vi "from string.vi"(8 "error in":errorcluster, 9 "data":string, 10 "version":string, 11 "Daqmx Module configuration in":refnum<class "DAQmx Module Configuration.lvclass">) -> (0 "error out":errorcluster, 3 "Daqmx Module configuration out":refnum<class "DAQmx Module Configuration.lvclass">)   [LabVIEW 2014, in "DAQmx Module Configuration.lvclass"]
doc: "Provides an interface for loading a module configuration from a file or other serialized data source. It is recommended that all children of this class store data in two sets--data required for its own initialization, and any data required for parent initialization--and that each implementation uses the <b>Call Parent Method</b> primitive to de-serialize parent information. As a result, it is expected that every module configuration class calls <b>component configuration.lvclass:From String.vi</b>."
uses:
  DAQmx Module Configuration.lvclass
  Line.ctl
  <vilib>/NI/Tag Bus Module Framework/channel/TBM channel.lvclass
  Measurement Type.ctl
  Parameters.ctl
  DAQmx Module Configuration.lvclass/DAQmx Module Configuration.ctl
  <vilib>/NI/Tag Bus Module Framework/module configuration/TBM module configuration.lvclass
  <vilib>/NI/Configuration Framework/serializable configuration/NISE_CEF_serializable configuration.lvclass
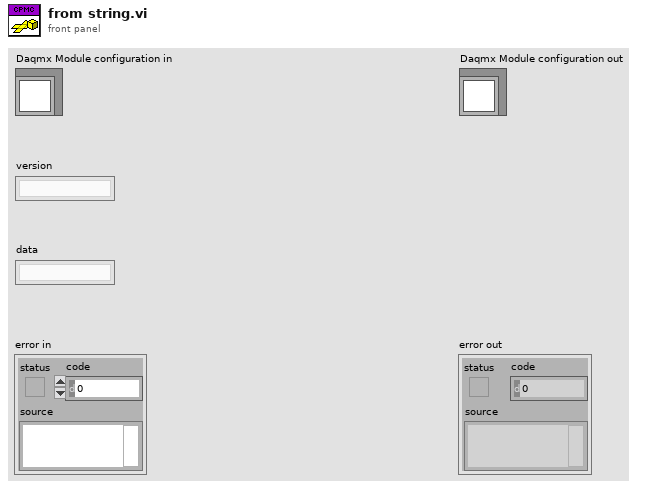
[diagram p1: front panel]
types:
  T1 = typedef "DAQmx Module Configuration.lvclass/Line.ctl" = cluster{"channel":refnum<class "TBM channel.lvclass">, "Physical Channel":string, "Measurement Type":T2, "Parameters":T3}
  T2 = typedef "DAQmx Module Configuration.lvclass/Measurement Type.ctl" = enum16{"Digital Input", "Digital Output", "Voltage Input", "Voltage Output", "Current Input", "Current Output", "RTD", "Thermocouple", "Strain"}
  T3 = typedef "DAQmx Module Configuration.lvclass/Parameters.ctl" = cluster{"Digital Config":cluster{"Invert Lines?":bool}, "Voltage Config":cluster{"Maximum Value (V)":dbl, "Minimum Value (V)":dbl, "in terminal configuration (V)":i32, "out terminal configuration (V)":i32}, "Current Config":cluster{"Maximum Value (A)":dbl, "Minimum Value (A)":dbl, "shunt resistor location":i32, "input terminal configuration (C)":i32, "external shunt resistor value":dbl}, "RTD Config":cluster{"Maximum Value (°C)":dbl, "Minimum Value (°C)":dbl, "resistance configuration":i32, "r0":dbl, "current excitation value":dbl, "rtd type":i32, "current excitation source":i32}, "Thermocouple Config":cluster{"Minimum Value (C)":dbl, "Maximum Value (C)":dbl, "thermocouple type":i32, "cjc source":i32, "cjc value":dbl}, "Strain Config":cluster{"Maximum Value":dbl, "Minimum Value":dbl, "bridge information":cluster{"strain configuration":i32, "lead wire resistance":dbl, "initial bridge voltage":dbl, "voltage excitation source":i32, "voltage excitation value":dbl}, "strain gage information":cluster{"gage factor":dbl, "nominal gage resistance":dbl, "poisson ratio":dbl}}}
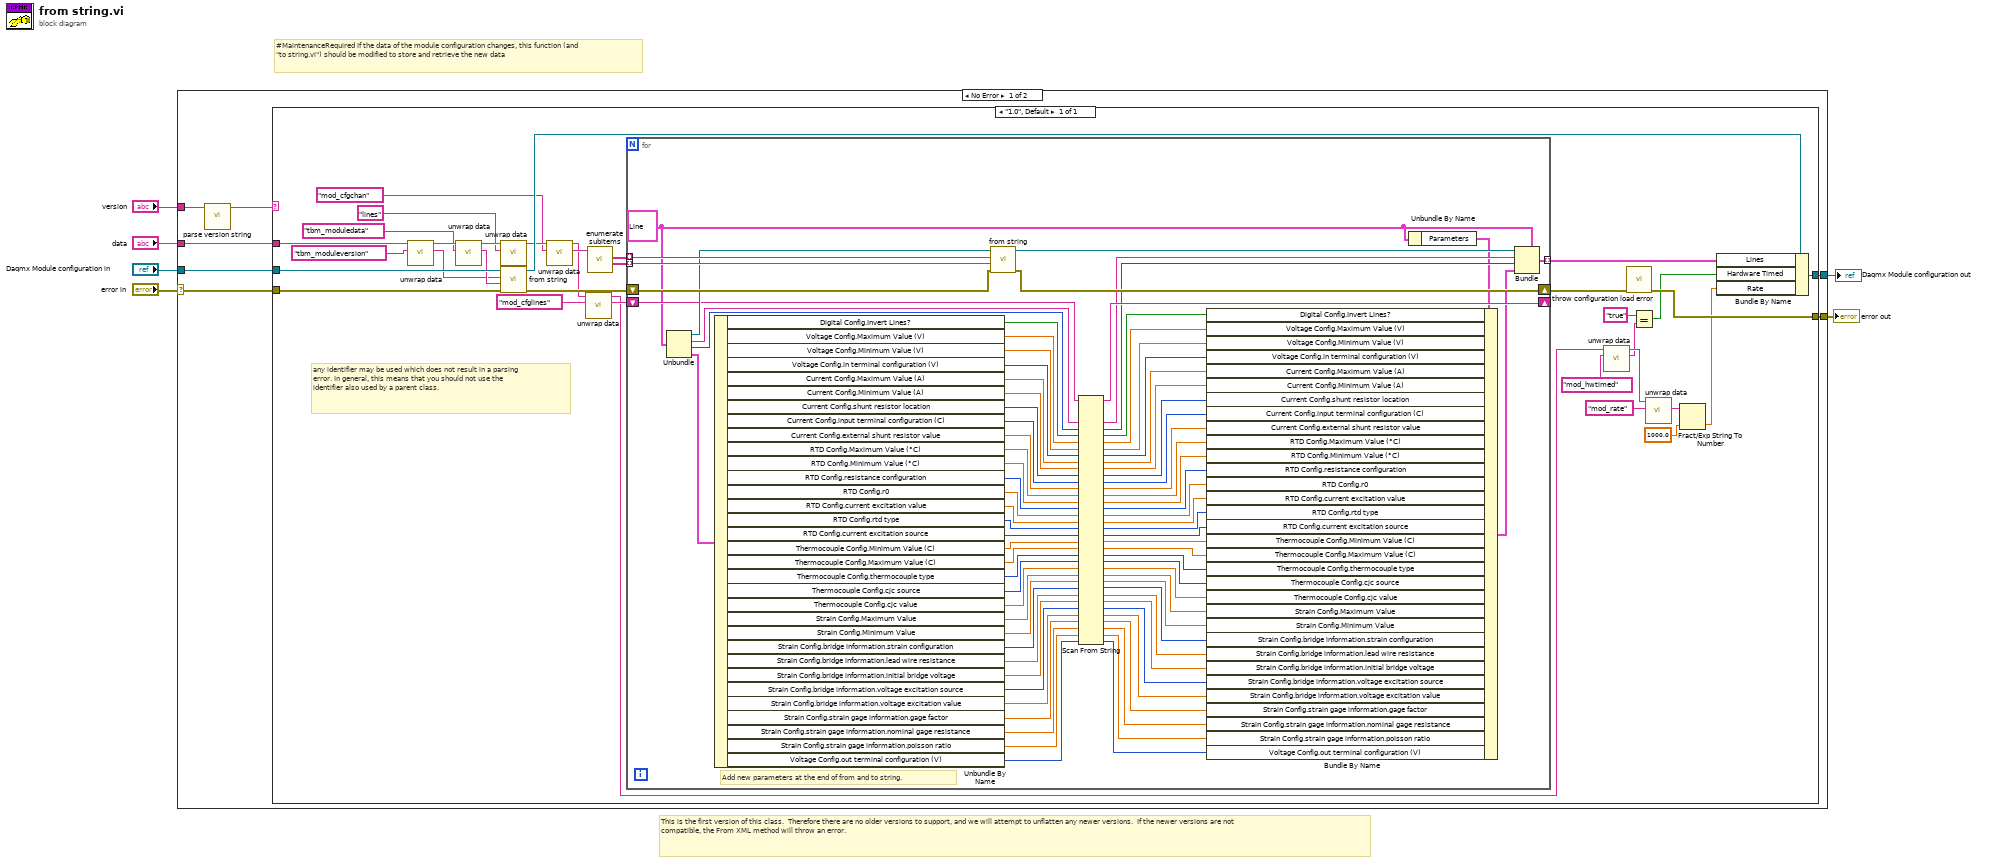
[diagram p0: block diagram]
diagram:
  # "#MaintenanceRequired If the data of the module configuration changes, this function (and \"to string.vi\") should be modified to store and retrieve the new data"
  # "This is the first version of this class.  Therefore there are no older versions to support, and we will attempt to unflatten any newer versions.  If the newer versions are not compatible, the From XML method will throw an error."
  n1 = case shown="No Error" "error in" {
    selector: "error in" -> [w7 w130]
    tunnel: "data" -> [w13 _]
    tunnel: "Daqmx Module configuration in" -> [w12 w129]
    tunnel: [w11 w129] -> w1
    tunnel: [w10 w130] -> w6
    tunnel: "version" -> [w9 _]
    frame No Error {
      n2 = call <vilib>:"parse version string.vi"("full version"=w9) -> ("major.minor version"=w8:string)  [unwired: 7 in, 3 out]
      n3 = case shown="\"1.0\", Default" w8 {
        tunnel: w13 -> [w44]
        tunnel: w7 -> [w43]
        tunnel: w12 -> [w47]
        tunnel: [w35] -> w11
        tunnel: [w46] -> w10
        frame "1.0", Default {
          # "any identifier may be used which does not result in a parsing error. In general, this means that you should not use the identifier also used by a parent class."
          n4 = call <vilib>:"unwrap data.vi"("identifier"="tbm_moduleversion" ("additional identifier"), "data to unwrap"=w44) -> ("unwrapped data"=w39:string, "remaining string"=w45:string)  [unwired: 8 in]
          n5 = call <vilib>:"unwrap data.vi"("identifier"="tbm_moduledata" ("additional identifier"), "data to unwrap"=w45) -> ("unwrapped data"=w41:string, "remaining string"=w38:string)  [unwired: 8 in]
          n6 = call <vilib>:"unwrap data.vi"("identifier"="lines" ("additional identifier"), "data to unwrap"=w38) -> ("remaining string"=w34:string)  [unwired: 8 in, 1 out]
          n7 = call-parent "from string.vi"("error in"=w43, "data"=w41, "version"=w39, "module configuration in"=w47) -> ("error out"=w30:errorcluster, "module configuration out"=w36:refnum<class "DAQmx Module Configuration.lvclass">)  [unwired: 6 in]
          n8 = call <vilib>:"unwrap data.vi"("identifier"="mod_cfgchan", "data to unwrap"=w34) -> ("unwrapped data"=w29:string, "remaining string"=w26:string)  [unwired: 8 in]
          n9 = call <vilib>:"unwrap data.vi"("identifier"="mod_cfglines", "data to unwrap"=w26) -> ("unwrapped data"=w24:string, "remaining string"=w14:string)  [unwired: 8 in]
          n10 = call <vilib>:"enumerate subitems.vi"("data to enumerate"=w29) -> ("associated data"=w31:string[], "discovered subitems"=w32:string[])  [unwired: 8 in, 1 out]
          n11 = for {
            shift-right: [w123] -> w28
            shift-left: w30 -> [w128]
            tunnel: w32 -> [w127] mode=indexing
            tunnel: w31 -> [w126] mode=indexing
            tunnel: [w124] -> w27 mode=indexing
            shift-right: [w95] -> _
            shift-left: w24 -> [w96]
            w51 = T1 {"channel"=refnum, "Physical Channel"="", "Measurement Type"=enum."Digital Input", "Parameters"={"Digital Config"={"Invert Lines?"=FALSE}, "Voltage Config"={"Maximum Value (V)"=5.0, "Minimum Value (V)"=-5.0, "in terminal configuration (V)"=-1, "out terminal configuration (V)"=-1}, "Current Config"={"Maximum Value (A)"=0.02, "Minimum Value (A)"=0.0, "shunt resistor location"=-1, "input terminal configuration (C)"=-1, "external shunt resistor value"=249.0}, "RTD Config"={"Maximum Value (°C)"=100.0, "Minimum Value (°C)"=0.0, "resistance configuration"=2, "r0"=100.0, "current excitation value"=0.0025, "rtd type"=10137, "current excitation source"=10167}, "Thermocouple Config"={"Minimum Value (C)"=0.0, "Maximum Value (C)"=100.0, "thermocouple type"=10072, "cjc source"=10116, "cjc value"=25.0}, "Strain Config"={"Maximum Value"=0.001, "Minimum Value"=-0.001, "bridge information"={"strain configuration"=10183, "lead wire resistance"=0.0, "initial bridge voltage"=0.0, "voltage excitation source"=10200, "voltage excitation value"=2.5}, "strain gage information"={"gage factor"=2.0, "nominal gage resistance"=350.0, "poisson ratio"=0.3}}}} ("Line")
            # "Add new parameters at the end of from and to string."
            n12 = Unbundle(w51) -> ("channel"=w122:refnum<class "TBM channel.lvclass">, "Physical Channel"=w121:string, "Measurement Type"=w97:T2, "Parameters"=w93:T3)
            n13 = Unbundle By Name(w93) -> ("Digital Config.Invert Lines?"=w120:bool, "Voltage Config.Maximum Value (V)"=w119:dbl, "Voltage Config.Minimum Value (V)"=w118:dbl, "Voltage Config.in terminal configuration (V)"=w117:i32, "Current Config.Maximum Value (A)"=w116:dbl, "Current Config.Minimum Value (A)"=w115:dbl, "Current Config.shunt resistor location"=w114:i32, "Current Config.input terminal configuration (C)"=w113:i32, "Current Config.external shunt resistor value"=w111:dbl, "RTD Config.Maximum Value (°C)"=w112:dbl, "RTD Config.Minimum Value (°C)"=w110:dbl, "RTD Config.resistance configuration"=w109:i32, "RTD Config.r0"=w108:dbl, "RTD Config.current excitation value"=w107:dbl, "RTD Config.rtd type"=w106:i32, "RTD Config.current excitation source"=w105:i32, "Thermocouple Config.Minimum Value (C)"=w104:dbl, "Thermocouple Config.Maximum Value (C)"=w103:dbl, "Thermocouple Config.thermocouple type"=w102:i32, "Thermocouple Config.cjc source"=w101:i32, "Thermocouple Config.cjc value"=w100:dbl, "Strain Config.Maximum Value"=w99:dbl, "Strain Config.Minimum Value"=w98:dbl, "Strain Config.bridge information.strain configuration"=w92:i32, "Strain Config.bridge information.lead wire resistance"=w91:dbl, "Strain Config.bridge information.initial bridge voltage"=w90:dbl, "Strain Config.bridge information.voltage excitation source"=w89:i32, "Strain Config.bridge information.voltage excitation value"=w88:dbl, "Strain Config.strain gage information.gage factor"=w87:dbl, "Strain Config.strain gage information.nominal gage resistance"=w86:dbl, "Strain Config.strain gage information.poisson ratio"=w85:dbl, "Voltage Config.out terminal configuration (V)"=w49:i32)
            n14 = call-dynamic "from string.vi"("error in"=w128, "channel data"=w126, "identifier"=w127, "channel in"=w122) -> ("error out"=w123:errorcluster, "channel out"=w125:refnum<class "TBM channel.lvclass">)  [unwired: 6 in]
            n15 = Scan From String(input string=w96, default 1=w121, default 2=w97, default 3=w120, default 4=w119, default 5=w118, default 6=w117, default 7=w116, default 8=w115, default 9=w114, default 10=w113, default 11=w111, default 12=w112, default 13=w110, default 14=w109, default 15=w108, default 16=w107, default 17=w106, default 18=w105, default 19=w104, default 20=w103, default 21=w102, default 22=w101, default 23=w100, default 24=w99, default 25=w98, default 26=w92, default 27=w91, default 28=w90, default 29=w89, default 30=w88, default 31=w87, default 32=w86, default 33=w85, default 34=w49) -> (remaining string=w95:string, output 1=w94:string, output 2=w84:T2, output 3=w83:bool, output 4=w82:dbl, output 5=w81:dbl, output 6=w80:i32, output 7=w79:dbl, output 8=w78:dbl, output 9=w77:i32, output 10=w76:i32, output 11=w75:dbl, output 12=w74:dbl, output 13=w73:dbl, output 14=w72:i32, output 15=w71:dbl, output 16=w70:dbl, output 17=w69:i32, output 18=w68:i32, output 19=w67:dbl, output 20=w66:dbl, output 21=w65:i32, output 22=w64:i32, output 23=w63:dbl, output 24=w62:dbl, output 25=w61:dbl, output 26=w60:i32, output 27=w59:dbl, output 28=w58:dbl, output 29=w57:i32, output 30=w56:dbl, output 31=w55:dbl, output 32=w54:dbl, output 33=w53:dbl, output 34=w48:i32)  [unwired: 3 in, 2 out]
            n16 = Unbundle By Name(w51) -> ("Parameters"=w50:T3)
            n17 = Bundle By Name(cluster=w50, "Digital Config.Invert Lines?"=w83, "Voltage Config.Maximum Value (V)"=w82, "Voltage Config.Minimum Value (V)"=w81, "Voltage Config.in terminal configuration (V)"=w80, "Current Config.Maximum Value (A)"=w79, "Current Config.Minimum Value (A)"=w78, "Current Config.shunt resistor location"=w77, "Current Config.input terminal configuration (C)"=w76, "Current Config.external shunt resistor value"=w75, "RTD Config.Maximum Value (°C)"=w74, "RTD Config.Minimum Value (°C)"=w73, "RTD Config.resistance configuration"=w72, "RTD Config.r0"=w71, "RTD Config.current excitation value"=w70, "RTD Config.rtd type"=w69, "RTD Config.current excitation source"=w68, "Thermocouple Config.Minimum Value (C)"=w67, "Thermocouple Config.Maximum Value (C)"=w66, "Thermocouple Config.thermocouple type"=w65, "Thermocouple Config.cjc source"=w64, "Thermocouple Config.cjc value"=w63, "Strain Config.Maximum Value"=w62, "Strain Config.Minimum Value"=w61, "Strain Config.bridge information.strain configuration"=w60, "Strain Config.bridge information.lead wire resistance"=w59, "Strain Config.bridge information.initial bridge voltage"=w58, "Strain Config.bridge information.voltage excitation source"=w57, "Strain Config.bridge information.voltage excitation value"=w56, "Strain Config.strain gage information.gage factor"=w55, "Strain Config.strain gage information.nominal gage resistance"=w54, "Strain Config.strain gage information.poisson ratio"=w53, "Voltage Config.out terminal configuration (V)"=w48) -> (w52:T3)
            n18 = Bundle(cluster=w51, "channel"=w125, "Physical Channel"=w94, "Measurement Type"=w84, "Parameters"=w52) -> (w124:T1)
          }
          n19 = call <vilib>:"unwrap data.vi"("identifier"="mod_hwtimed", "data to unwrap"=w14) -> ("unwrapped data"=w20:string, "remaining string"=w21:string)  [unwired: 8 in]
          n20 = call <vilib>:"throw configuration load error.vi"("error in"=w28) -> ("error out"=w46:errorcluster)  [unwired: 10 in]
          n21 = Equal?(x="true" ("identifier"), y=w20) -> (x = y?=w18:bool)
          n22 = call <vilib>:"unwrap data.vi"("identifier"="mod_rate", "data to unwrap"=w21) -> ("unwrapped data"=w17:string)  [unwired: 8 in, 1 out]
          n23 = Fract/Exp String To Number(string=w17, default (0 dbl)=1000.0 ("default (0 DBL)")) -> (number=w16:dbl)  [unwired: 2 in, 1 out]
          n24 = Bundle By Name(cluster=w36, "Lines"=w27, "Hardware Timed"=w18, "Rate"=w16) -> (w35:refnum<class "DAQmx Module Configuration.lvclass">)
        }
      }
    }
    frame Error {
    }
  }
  "error out" <- w6
  "Daqmx Module configuration out" <- w1
